vi "LEP_RV_WriteSymbolDataToXML.vi"(8 "error in":errorcluster, 10 "XML file refnum":refnum<file>, 11 "Symbol elements array":string[](array[string])) -> (0 "error out":errorcluster)   [LabVIEW 2011]
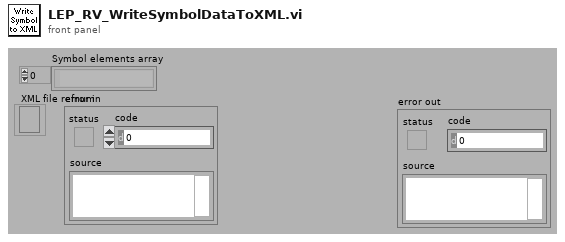
[diagram p1: front panel]
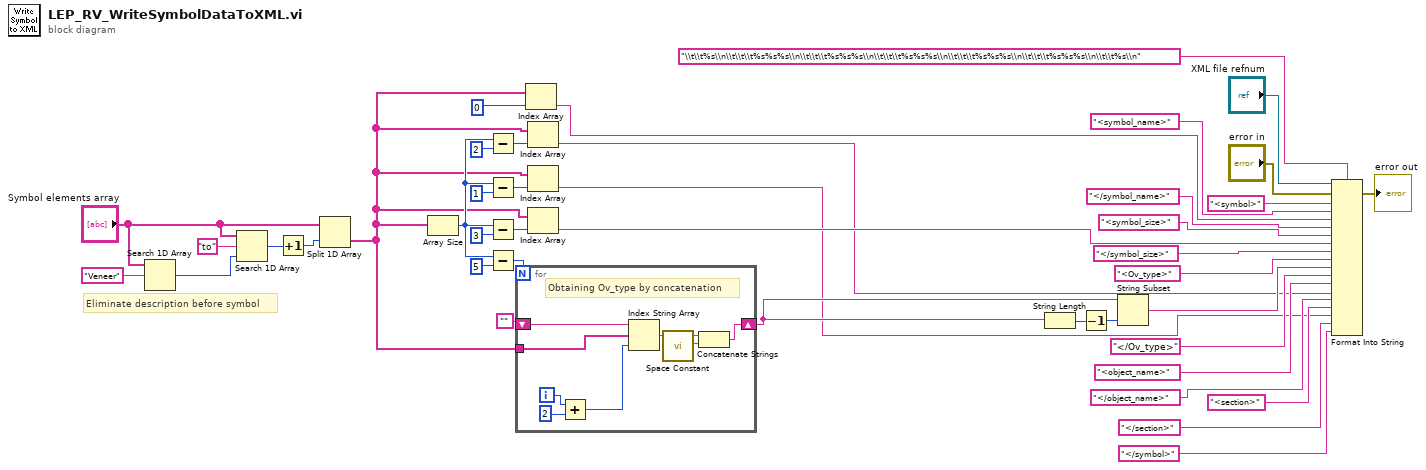
[diagram p0: block diagram]
diagram:
  # "Eliminate description before symbol"
  n1 = Search 1D Array(1D array="Symbol elements array", element="Veneer") -> (index of element=w5:i32)  [unwired: 1 in]
  n2 = Search 1D Array(1D array="Symbol elements array", element="to", start index (0)=w5) -> (index of element=w2:i32)
  n3 = Increment(x=w2) -> (x+1=w1:i32)
  n4 = Split 1D Array(array="Symbol elements array", index=w1) -> (second subarray=w3:string[])  [unwired: 1 out]
  n5 = Array Size(array=w3) -> (size(s)=w13:i32)
  n6 = Subtract(x=w13, y=2) -> (x-y=w20:i32)
  n7 = Subtract(x=w13, y=1) -> (x-y=w15:i32)
  n8 = Subtract(x=w13, y=3) -> (x-y=w32:i32)
  n9 = Subtract(x=w13, y=5) -> (x-y=w28:i32)
  n10 = for "Obtaining Ov_type by concatenation" {
    N: w28 -> [_]
    tunnel: w3 -> [w47]
    shift-right: [w46] -> w24
    shift-left: "" -> [w45]
    i -> [w50]
    # "Obtaining Ov_type by concatenation"
    n11 = Add(x=w50, y=2) -> (x+y=w48:i32)
    n12 = Index String Array(1:w48, 2:w47, 3:w45) -> (0:w44:string)
    n13 = call <vilib>:"Space Constant.vi"() -> ("String"=w43:string)
    n14 = Concatenate Strings(w44, w43) -> (w46:string)
  }
  n15 = Index Array(array=w3, index=0) -> (element=w38:string)
  n16 = Index Array(array=w3, index=w20) -> (element=w18:string)
  n17 = Index Array(array=w3, index=w15) -> (element=w8:string)
  n18 = Index Array(array=w3, index=w32) -> (element=w34:string)
  n19 = String Length(string=w24) -> (length=w26:i32)
  n20 = Decrement(x=w26) -> (x-1=w25:i32)
  n21 = String Subset(string=w24, length (rest)=w25) -> (substring=w23:string)  [unwired: 1 in]
  n22 = Format Into String(format string="\\t\\t%s\\n\\t\\t\\t%s%s%s\\n\\t\\t\\t%s%s%s\\n\\t\\t\\t%s%s%s\\n\\t\\t\\t%s%s%s\\n\\t\\t\\t%s%s%s\\n\\t\\t%s\\n", initial string="XML file refnum", error in="error in", "<symbol>" ("input 1"), "<symbol_name>" ("input 2"), w38, "</symbol_name>" ("input 3"), "<symbol_size>" ("input 5"), w34, "</symbol_size>" ("input 7"), "<Ov_type>" ("input 8"), w23, "</Ov_type>" ("input 10"), "<object_name>" ("input 11"), w18, "</object_name>" ("input 13"), "<section>" ("input 14"), w8, "</section>" ("input 16"), "</symbol>" ("input 17")) -> (error out=→"error out":errorcluster)  [unwired: 1 out]
